vi "_RT_CtrlLoop_Pub_Wfm_ScanData.vi"(7 "Function":T1=enum."Set", 8 "error in (no error)":errorcluster, 10 "WFM_U64Arr in":u64[](array[numeric])) -> (0 "error out":errorcluster, 2 "WFM_U64Arr out":u64[](array[numeric]))   [LabVIEW 2018]
uses:
  Ctl/_ctl_Integrated_Cmd.ctl
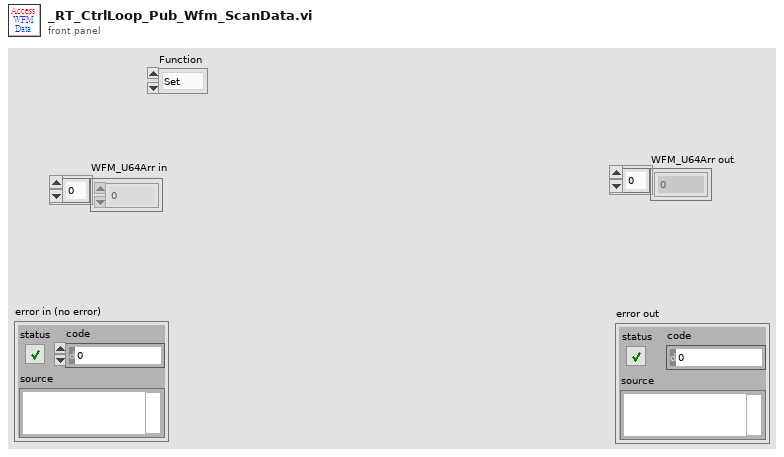
[diagram p1: front panel]
types:
  T1 = typedef "_ctl_Integrated_Cmd.ctl" = enum8{"Init", "Set", "Get", "Read", "Write", "Send", "Idle", "Startup", "Execution", "End", "Close"}
  T2 = enum16{"open", "replace", "create", "open or create", "replace or create", "replace or create with confirmation"}
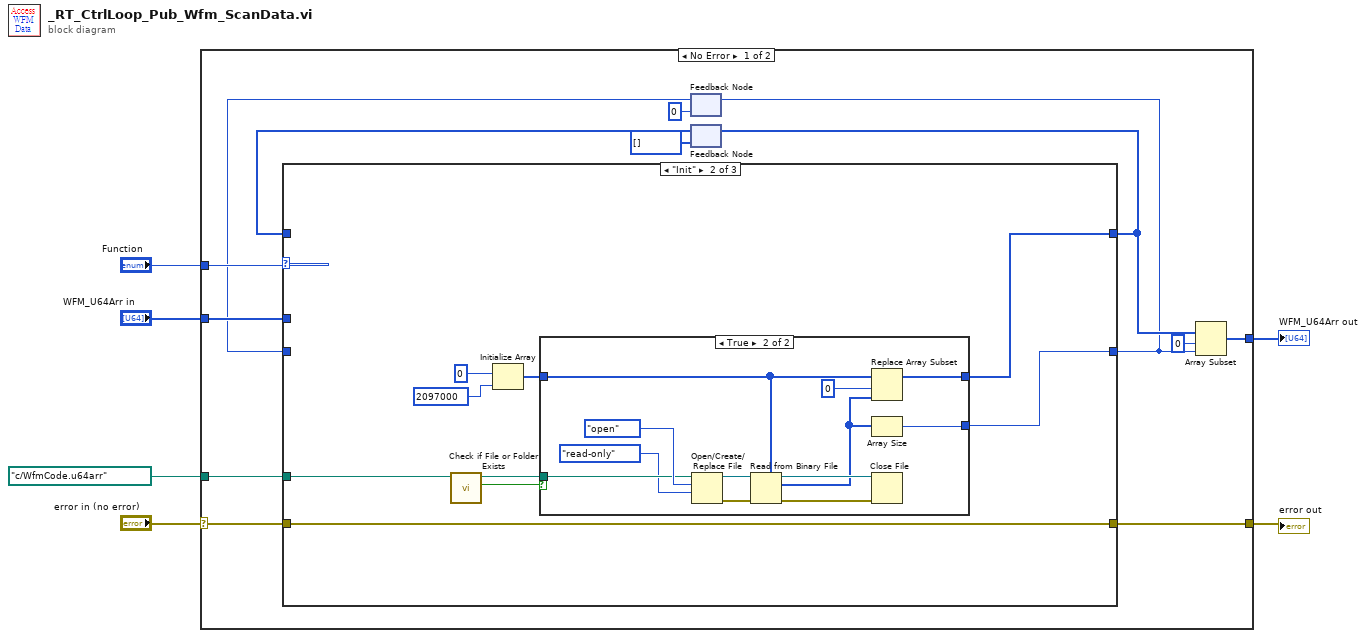
[diagram p0: block diagram]
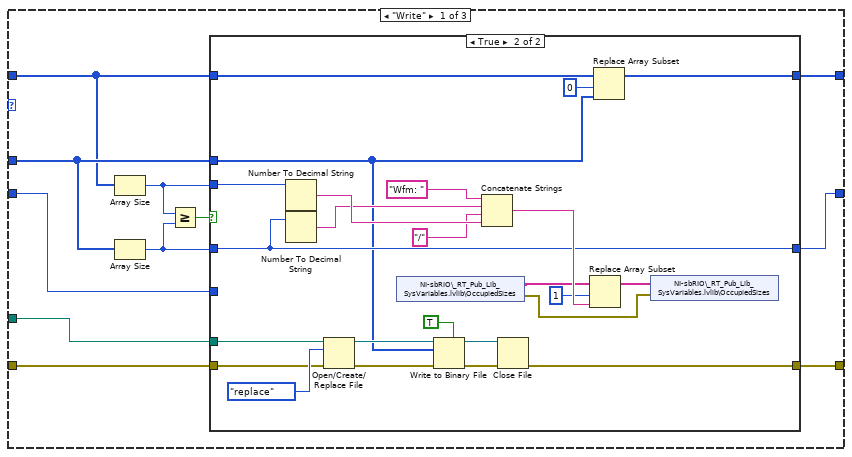
[diagram p2: hidden frame]
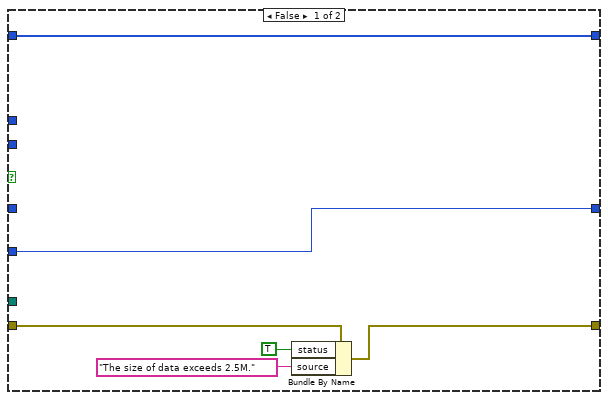
[diagram p3: hidden frame]
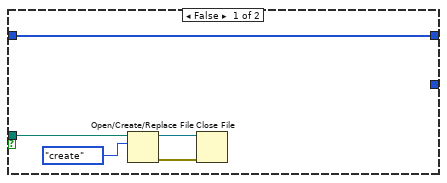
[diagram p4: hidden frame]
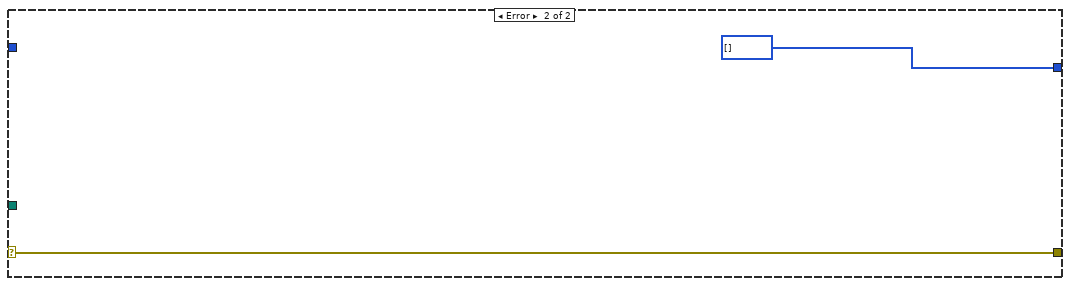
[diagram p6: hidden frame]
diagram:
  n1 = case shown="No Error" "error in (no error)" {
    selector: "error in (no error)" -> [w16 w91]
    tunnel: "Function" -> [w19 _]
    tunnel: "WFM_U64Arr in" -> [w18 _]
    tunnel: [w15 w91] -> w4
    tunnel: [w10 u64[] []] -> w3
    tunnel: path "c:/WfmCode.u64arr" ("file path (use dialog)") -> [w9 _]
    frame No Error {
      n2 = feedback #1(0) -> (w14:i32)
      n3 = feedback #2(u64[] []) -> (w17:u64[])
      n4 = case shown="\"Init\"" w19 {
        tunnel: w18 -> [w29 _ _]
        tunnel: [w30 w63 w89] -> w13
        tunnel: w17 -> [w27 _ w89]
        tunnel: w16 -> [w26 w67 w88]
        tunnel: [w25 w67 w88] -> w15
        tunnel: [w23 w62 w87] -> w12
        tunnel: w14 -> [w22 _ w87]
        tunnel: w9 -> [w20 w61 _]
        frame "Write" {
          n5 = Array Size(array=w27) -> (size(s)=w21:i32)
          n6 = Array Size(array=w29) -> (size(s)=w24:i32)
          n7 = Greater Or Equal?(x=w21, y=w24) -> (x >= y?=w28:bool)
          n8 = case shown="True" w28 {
            tunnel: w27 -> [w36 w60]
            tunnel: [w36 w59] -> w30
            tunnel: w29 -> [_ w40]
            tunnel: w26 -> [w35 w37]
            tunnel: [w32 w38] -> w25
            tunnel: w24 -> [_ w48]
            tunnel: [w31 w48] -> w23
            tunnel: w22 -> [w31 _]
            tunnel: w21 -> [_ w49]
            tunnel: w20 -> [_ w39]
            frame False {
              n9 = Bundle By Name(cluster=w35, "status"=TRUE, "source"="The size of data exceeds 2.5M.") -> (w32:errorcluster)
            }
            frame True {
              n10 = Number To Decimal String(number=w49) -> (decimal integer string=w53:string)  [unwired: 1 in]
              n11 = Number To Decimal String(number=w48) -> (decimal integer string=w52:string)  [unwired: 1 in]
              n12 = Open/Create/Replace File(file path (use dialog)=w39, error in=w37, operation (0:open)=T2."replace") -> (refnum out=w45:refnum<file>, error out=w44:errorcluster)  [unwired: 3 in, 1 out]
              n13 = shared-variable "NI-sbRIO\\_RT_Pub_Lib_SysVariables.lvlib\\OccupiedSizes"() -> (w56:string[], error out=w47:errorcluster)  [unwired: 1 in]
              n14 = Write to Binary File(file (use dialog)=w45, data=w40, error in=w44, 5:TRUE ("prepend array or string size? (T)")) -> (refnum out=w42:refnum<file>, error out=w41:errorcluster)  [unwired: 2 in, 1 out]
              n15 = Concatenate Strings("Wfm: " ("element"), w52, "/" ("element"), w53) -> (w57:string)
              n16 = Close File(refnum=w42, error in=w41) -> (error out=w38:errorcluster)  [unwired: 1 out]
              n17 = Replace Array Subset(array=w56, new element=w57, index=1) -> (w54:string[])
              n18 = Replace Array Subset(array=w60, new element=w40, index=0) -> (w59:u64[])
              n19 = shared-variable "NI-sbRIO\\_RT_Pub_Lib_SysVariables.lvlib\\OccupiedSizes"(w54, error in=w47) -> ()  [unwired: 1 out]
            }
          }
        }
        frame "Init" {
          n20 = call <vilib>:"Check if File or Folder Exists.vi"("path"=w61) -> ("file or folder exists?"=w65:bool, "dup path"=w66:path)  [unwired: 8 in, 1 out]
          n21 = Initialize Array(u64 0, 2097000 ("dimension size")) -> (w64:u64[])
          n22 = case shown="True" w65 {
            tunnel: w66 -> [w73 w83]
            tunnel: w64 -> [w74 w79]
            tunnel: [w74 w77] -> w63
            tunnel: [_ w76] -> w62
            frame False {
              n23 = Open/Create/Replace File(file path (use dialog)=w73, operation (0:open)=T2."create") -> (refnum out=w71:refnum<file>, error out=w70:errorcluster)  [unwired: 4 in, 1 out]
              n24 = Close File(refnum=w71, error in=w70) -> ()  [unwired: 2 out]
            }
            frame True {
              n25 = Open/Create/Replace File(file path (use dialog)=w83, operation (0:open)=T2."open", access (0:read/write)=enum16{"read/write", "read-only", "write-only"}."read-only") -> (refnum out=w85:refnum<file>, error out=w84:errorcluster)  [unwired: 3 in, 1 out]
              n26 = Read from Binary File(5:w79, 8:w84, 11:w85) -> (0:w80:errorcluster, 2:w75:u64[], 3:w81:refnum<file>)  [unwired: 3 in, 1 out]
              n27 = Replace Array Subset(array=w79, new element=w75, index=0) -> (w77:u64[])
              n28 = Array Size(array=w75) -> (size(s)=w76:i32)
              n29 = Close File(refnum=w81, error in=w80) -> ()  [unwired: 2 out]
            }
          }
        }
        frame "Read", Default {
        }
      }
      n30 = feedback-in #1(w12) -> ()
      n31 = feedback-in #2(w13) -> ()
      n32 = Array Subset(array=w13, index=0, length=w12) -> (w10:u64[])
    }
    frame Error {
    }
  }
  "error out" <- w4
  "WFM_U64Arr out" <- w3
